vi "ExitConfirmation.vi"() -> (3 "Output":bool)   [LabVIEW 2018]
panel:
  in  "Cancel Button":bool
  in  "OK":bool
  # "Czy na pewno chcesz \n  zakoñczyæ trening?"
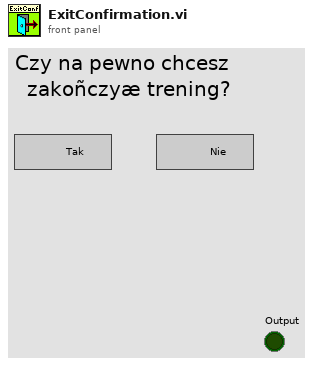
[diagram p1: front panel]
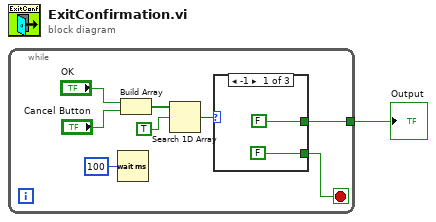
[diagram p0: block diagram]
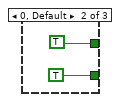
[diagram p2: hidden frame]
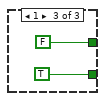
[diagram p3: hidden frame]
diagram:
  n1 = while {
    tunnel: [w2] -> w1
    stop <- w3 stop-if-true
    n2 = Wait (ms)(milliseconds to wait=u32 100) -> ()  [unwired: 1 out]
    n3 = Build Array("OK", "Cancel Button") -> (w6:bool[])
    n4 = Search 1D Array(1D array=w6, element=TRUE) -> (index of element=w4:i32)  [unwired: 1 in]
    n5 = case shown="-1" w4 {
      tunnel: [FALSE TRUE TRUE] -> w3
      tunnel: [FALSE TRUE FALSE] -> w2
      frame -1 {
      }
      frame 0, Default {
      }
      frame 1 {
      }
    }
  }
  "Output" <- w1
